vi "test_shuffle_array.vi"   [LabVIEW 2021]
uses:
  929d9f70-b382-3fdc-4057-ce21f6d5de3f.vi
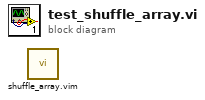
[diagram p0: block diagram]
diagram:
  n1 = call "shuffle_array.vim"() -> ()  [unwired: 1 in, 1 out]
